vi "niScope Self Test.vi"(0 "instrument handle":refnum<k15>, 11 "error in":errorcluster) -> (4 "instrument handle out":refnum<k15>, 6 "self-test message":string, 10 "self test result":i16 format="%.0x", 15 "error out":errorcluster)   [LabVIEW 2011]
doc: "Runs the device self-test routine and returns the test result(s)."
uses:
  niScope_32.dll
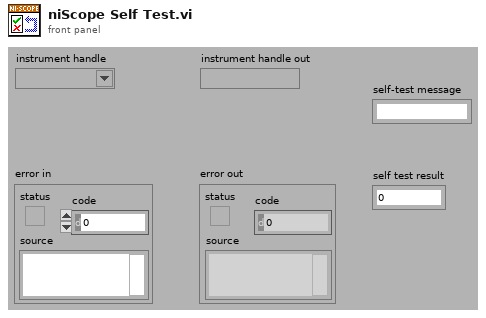
[diagram p1: front panel]
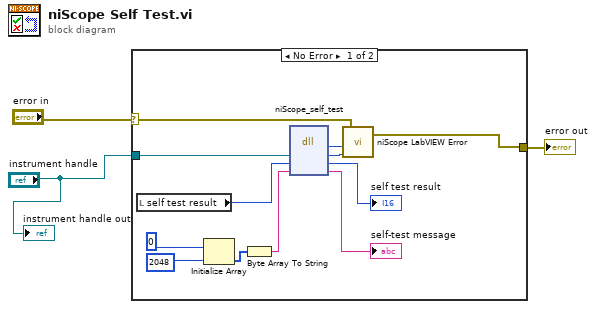
[diagram p0: block diagram]
diagram:
  n1 = case shown="No Error" "error in" {
    selector: "error in" -> [w4 w16]
    tunnel: [w5 w16] -> w3
    tunnel: "instrument handle" -> [w15 _]
    frame No Error {
      n2 = local read "self test result"() -> (w11:i16)
      n3 = Initialize Array(u8 0, 2048) -> (w12:u8[])
      n4 = Byte Array To String(unsigned byte array=w12) -> (string=w9:string)
      n5 = dll-call lib="niScope_*.*" fn="niScope_self_test"("instrument handle"=w15, "selfTestResult"=w11, "selfTestMessage"=w9) -> ("status"=w7:i32, "instrument handle"=w6:u32, "selfTestResult"=→"self test result":i16, "selfTestMessage"=→"self-test message":string)  [unwired: 3 in, 2 out]
      n6 = call <instrlib>:"niScope LabVIEW Error.vi"("instrument handle"=w6, "niScope error code (0)"=w7, "error in (no error)"=w4) -> ("error out"=w5:errorcluster)  [unwired: 2 in]
    }
    frame Error {
    }
  }
  "error out" <- w3
  "instrument handle out" <- "instrument handle"
